vi "Sequence.CreateMainSwitch.vi"(8 "error in (no error)":errorcluster) -> (0 "error out":errorcluster, 2 "Cases":refnum<k24>, 3 ".NET Refnum out":refnum<k24>)   [LabVIEW 2013, in "Simple Sequence Editor.lvlib"]
uses:
  Simple Sequence Editor.lvlib
  NationalInstruments.VeriStand.RealTimeSequenceDefinitionApi
  Constants.vi
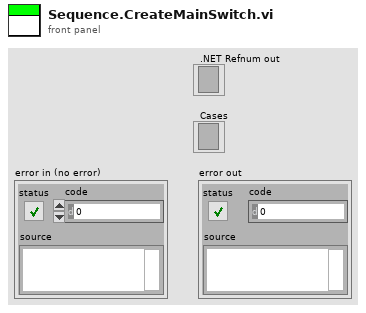
[diagram p1: front panel]
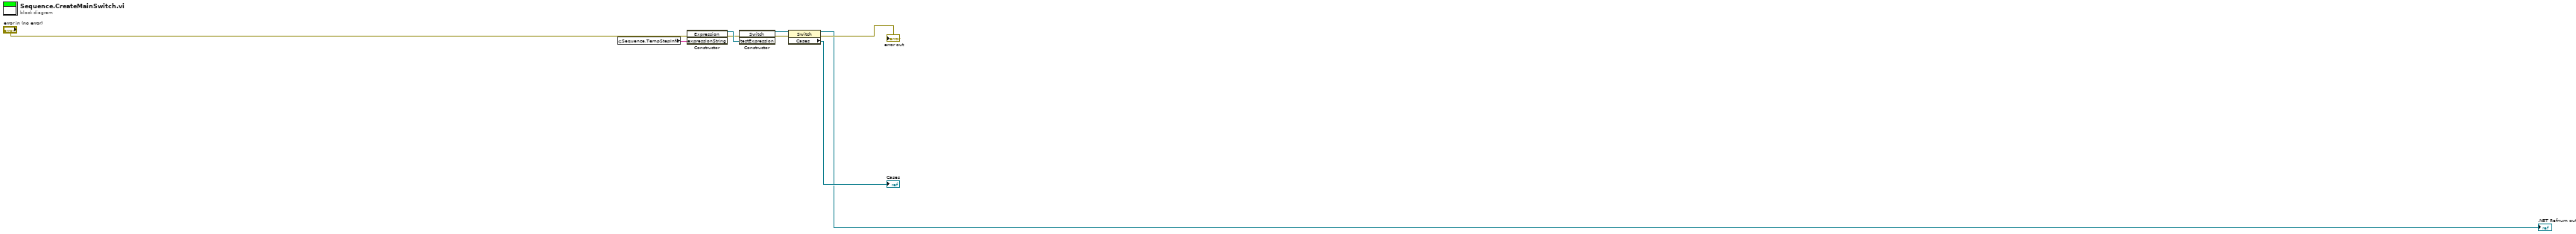
[diagram p0: block diagram]
diagram:
  n1 = global read "Constants.vi" "Sequence.TempStepInfo"() -> (w9:string)
  n2 = constructor class="Expression"(error in="error in (no error)", "expressionString"=w9) -> (reference out=w8:refnum<k24>, error out=w7:errorcluster)  [unwired: 2 in, 2 out]
  n3 = constructor class="Switch"(error in=w7, "testExpression"=w8) -> (reference out=w6:refnum<k24>, error out=w5:errorcluster)  [unwired: 2 in, 2 out]
  n4 = property class="Switch"(reference=w6, error in=w5) -> (reference out=→".NET Refnum out":refnum<k24>, error out=→"error out":errorcluster, "Cases"=→"Cases":refnum<k24>)
